vi "adaptive filter NLMS(sub VI).vi"(0 "ERR":dbl=0.060310676968585164, 1 "NLMS-r(防止過大步長)":dbl=10.0, 2 "輸入訊號":dbl, 3 "order":i32=10, 5 "u(收斂係數)":dbl=0.001) -> (6 "FIR輸出":dbl=-1.0516183080382016, 8 "權重":dbl[](array[numeric]))   [LabVIEW 2010]
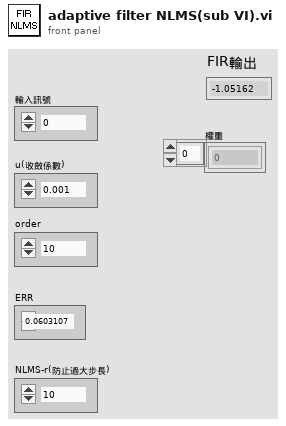
[diagram p1: front panel]
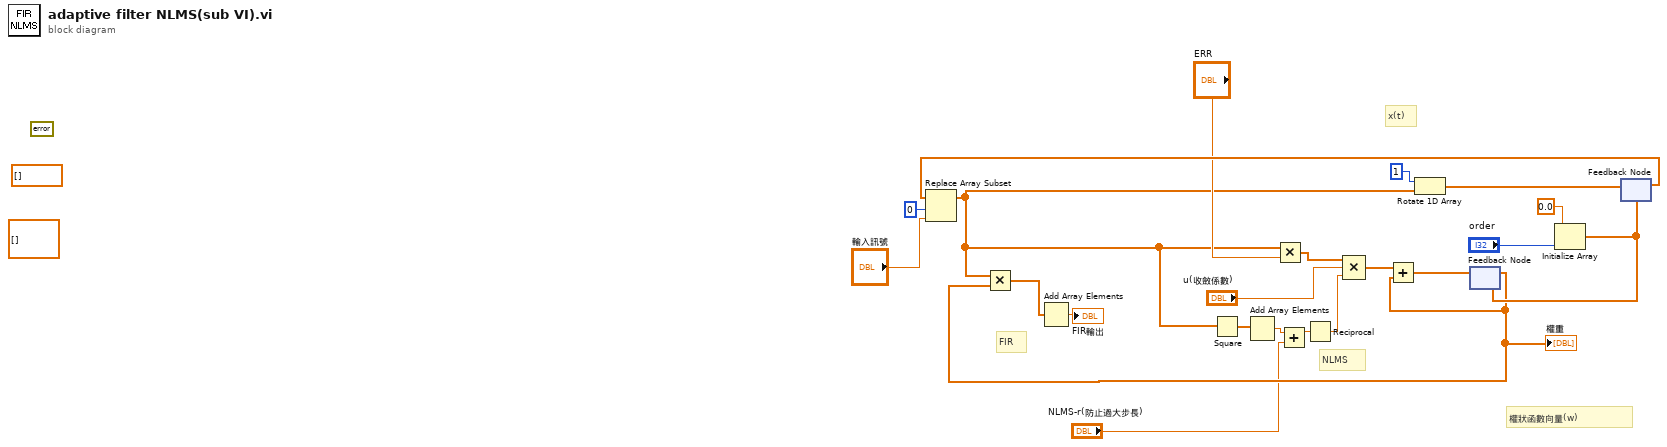
[diagram p0: block diagram]
diagram:
  (unwired) dbl[][] [] ("History Data")
  (unwired) dbl[] [] ("History Data")
  (unwired) errorcluster {"status"=FALSE, "code"=0, "source"=""} ("error constant")
  # "NLMS"
  # "FIR"
  # "權狀函數向量(w)"
  # "x(t)"
  n1 = Initialize Array(0.0 ("element"), "order") -> (w10:dbl[])
  n2 = feedback #1(w10) -> (w8:dbl[])
  "權重" <- w8
  n3 = feedback #2(w10) -> (w15:dbl[])
  n4 = Replace Array Subset(array=w15, new element="輸入訊號", index=0) -> (w7:dbl[])
  n5 = Multiply(x=w7, y=w8) -> (x*y=w18:dbl[])
  n6 = Add Array Elements(numeric array=w18) -> (sum=→"FIR輸出":dbl)
  n7 = Square(x=w7) -> (x^2=w6:dbl[])
  n8 = Add Array Elements(numeric array=w6) -> (sum=w5:dbl)
  n9 = Multiply(x=w7, y="ERR") -> (x*y=w22:dbl[])
  n10 = Add(x=w5, y="NLMS-r(防止過大步長)") -> (x+y=w3:dbl)
  n11 = Reciprocal(x=w3) -> (1/x=w1:dbl)
  n12 = Compound Arithmetic op=MULTIPLY(w22, "u(收斂係數)", w1) -> (w11:dbl[])
  n13 = Add(x=w11, y=w8) -> (x+y=w12:dbl[])
  n14 = Rotate 1D Array(1:w7, 2:1 ("n")) -> (0:w16:dbl[])
  n15 = feedback-in #1(w12) -> ()
  n16 = feedback-in #2(w16) -> ()
